vi "CSV_import_control_lasers_and_SMs_and_ICC4C.vi"() -> ()   [LabVIEW 2021]
uses:
  <vilib>/DAQmx/write.llb/DAQmx Write (Analog 1D DBL NChan 1Samp).vi
  <vilib>/DAQmx/create/channels.llb/DAQmx Create Channel (AO-Voltage-Basic).vi
  <vilib>/Utility/file.llb/Read Delimited Spreadsheet (DBL).vi
  <vilib>/DAQmx/miscellaneous.llb/DAQmx Fill In Error Info.vi
panel:
  out "Sequence Length":i32
  in  "Delay":i32
  in  "ICC4C 3 (0-10V)":dbl
  in  "ICC4C 2 (0-10V)":dbl
  in  "ICC4C 1 (0-10V)":dbl
  in  "ICC4C 0 (0-10V)":dbl
  in  "Y2 (-10-10V)":dbl
  in  "X2 (-10-10V)":dbl
  in  "Continue Cycle?":bool
  out "Full Cycles":i32
  out "Phase I Iterations":i32
  out "Y1 (-10-10V)":dbl format="%_6g"
  out "X1 (-10-10V)":dbl format="%_6g"
  in  "Blanking (0-10v)":dbl=10.0
  in  "561 (0-10v)":dbl
  in  "514 (0-10v)":dbl
  in  "488 (0-10v)":dbl
  in  "445 (0-10v)":dbl
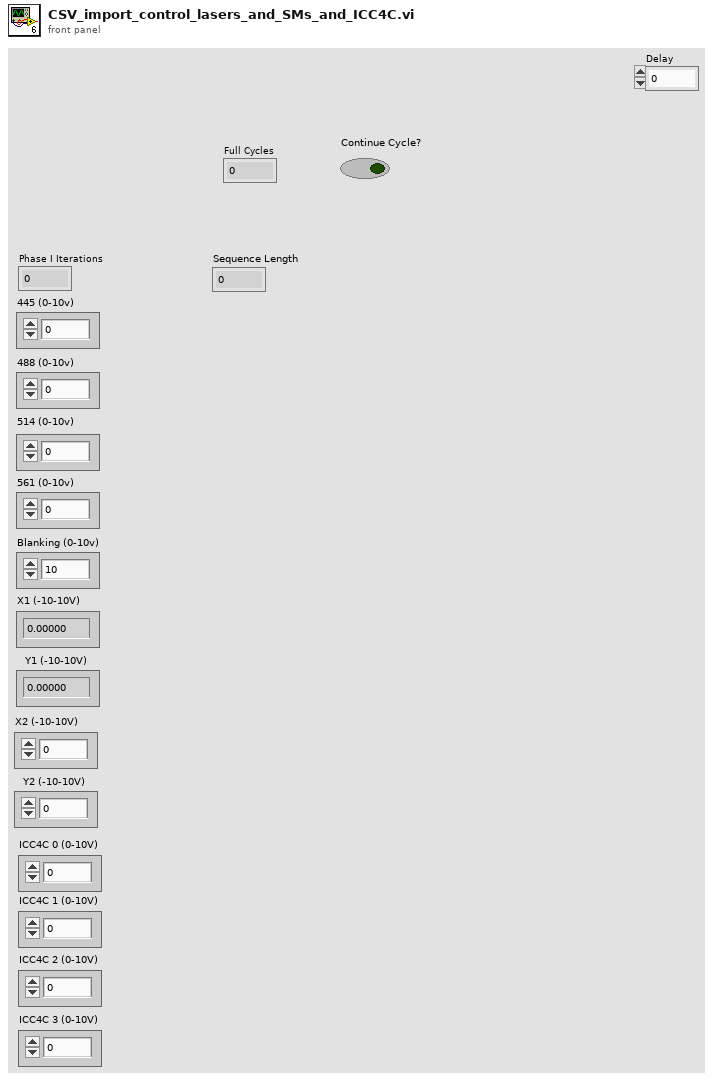
[diagram p1: front panel]
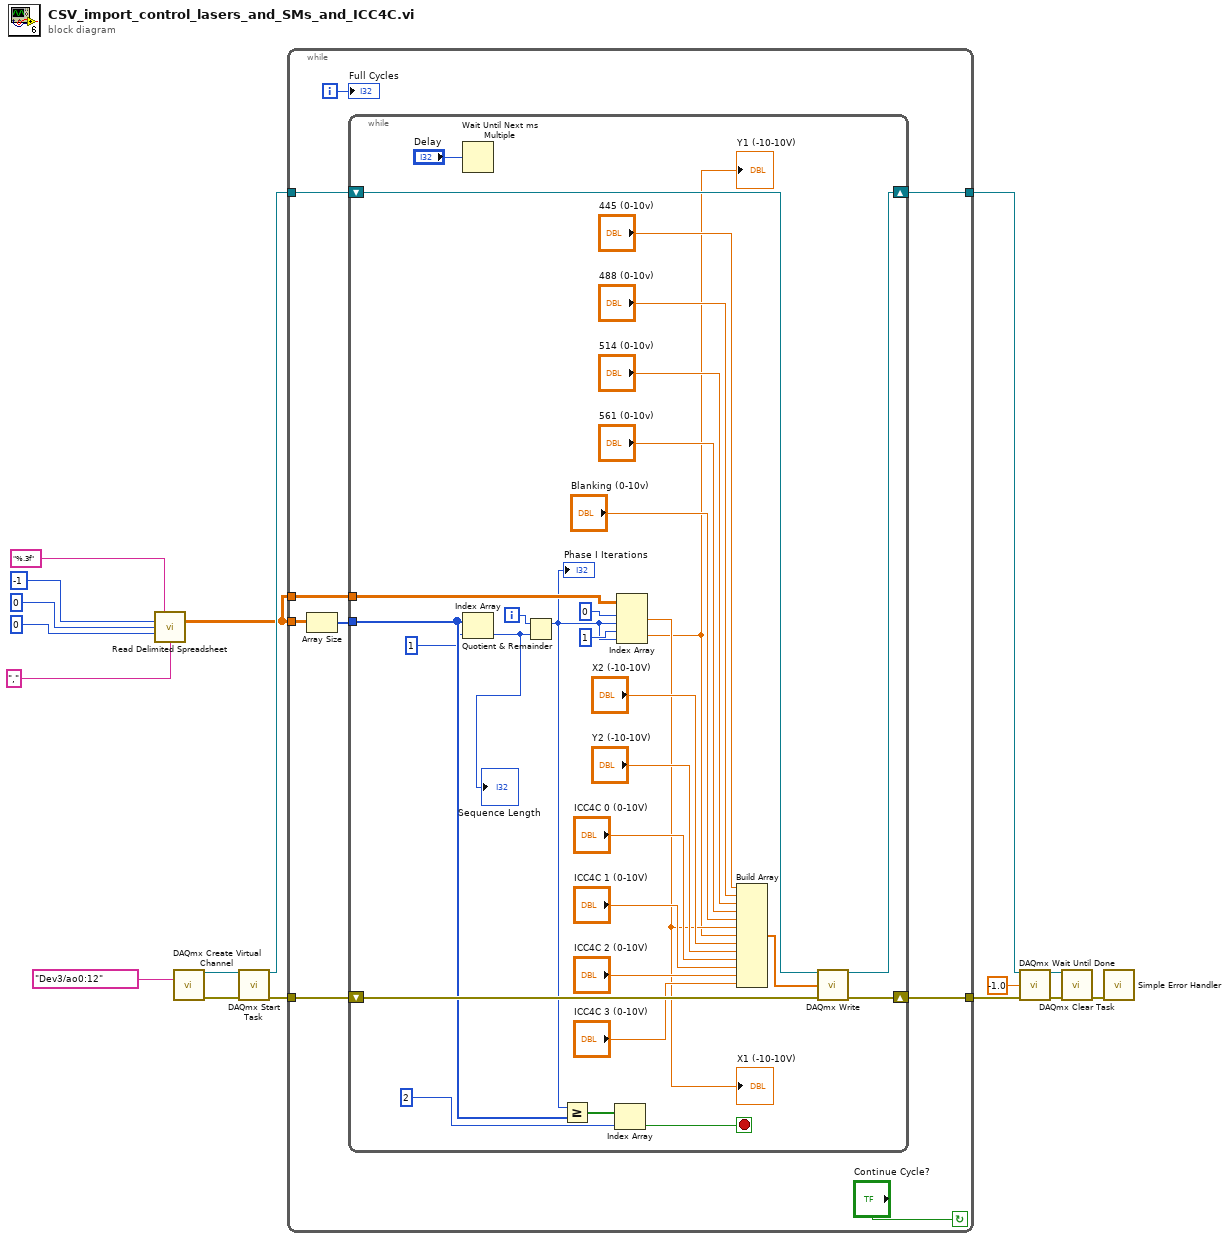
[diagram p0: block diagram]
diagram:
  n1 = call-poly <vilib>:"Read Delimited Spreadsheet.vi"("format (%.3f)"="%.3f", "number of rows (all:-1)"=-1, "start of read offset (chars.:0)"=0, "max characters/row  (no limit:0)"=0, "delimiter (\\t)"=",") -> ("all rows"=w6:dbl[][])  [unwired: 5 in, 5 out]
  n2 = call-poly <vilib>:"DAQmx Create Virtual Channel.vi"("physical channels"=tag "Dev3/ao0:12") -> ("task out"=w10:refnum<k21>, "error out"=w9:errorcluster)  [unwired: 13 in]
  n3 = call <vilib>:"DAQmx Start Task.vi"("task/channels in"=w10, "error in"=w9) -> ("task out"=w8:refnum<k21>, "error out"=w7:errorcluster)  [unwired: 12 in]
  n4 = while {
    tunnel: [w22] -> w13
    tunnel: [w21] -> w12
    tunnel: w8 -> [w25]
    tunnel: w7 -> [w24]
    tunnel: w6 -> [w19]
    tunnel: w6 -> [w18]
    i -> [w26]
    stop <- "Continue Cycle?" continue-if-true
    n5 = Array Size(array=w19) -> (size(s)=w20:i32[])
    n6 = while {
      shift-right: [w54] -> w22
      shift-left: w25 -> [w56]
      shift-right: [w53] -> w21
      shift-left: w24 -> [w55]
      tunnel: w20 -> [w31]
      tunnel: w18 -> [w36]
      i -> [w32]
      stop <- w37 stop-if-true
      n7 = Wait Until Next ms Multiple(millisecond multiple="Delay") -> ()  [unwired: 1 out]
      n8 = Index Array(array=w31, index=1) -> (element=w28:i32)
      "Sequence Length" <- w28
      n9 = Quotient & Remainder(x=w32, y=w28) -> (x-y*floor(x/y)=w29:i32)  [unwired: 1 out]
      "Phase I Iterations" <- w29
      n10 = Greater Or Equal?(x=w29, y=w31) -> (x >= y?=w38:bool[])
      n11 = Index Array(array=w38, index=2) -> (element=w37:bool)
      n12 = Index Array(array=w36, index (row) #1=0, index (col) #1=w29, index (row) #2=1, index (col) #2=w29) -> (element #1=w39:dbl, element #2=w35:dbl)
      "X1 (-10-10V)" <- w39
      "Y1 (-10-10V)" <- w35
      n13 = Build Array("445 (0-10v)", "488 (0-10v)", "514 (0-10v)", "561 (0-10v)", "Blanking (0-10v)", w39, w35, "X2 (-10-10V)", "Y2 (-10-10V)", "ICC4C 0 (0-10V)", "ICC4C 1 (0-10V)", "ICC4C 2 (0-10V)", "ICC4C 3 (0-10V)") -> (w52:dbl[])
      n14 = call-poly <vilib>:"DAQmx Write.vi"("task/channels in"=w56, "data"=w52, "error in"=w55) -> ("task out"=w54:refnum<k21>, "error out"=w53:errorcluster)  [unwired: 10 in, 1 out]
    }
    "Full Cycles" <- w26
  }
  n15 = call <vilib>:"DAQmx Wait Until Done.vi"("task/channels in"=w13, "timeout (sec)"=-1.0, "error in"=w12) -> ("task out"=w16:refnum<k21>, "error out"=w15:errorcluster)  [unwired: 11 in]
  n16 = call <vilib>:"DAQmx Clear Task.vi"("task in"=w16, "error in"=w15) -> ("error out"=w17:errorcluster)  [unwired: 13 in]
  n17 = call <vilib>:"Simple Error Handler.vi"("error in (no error)"=w17) -> ()  [unwired: 4 in, 5 out]
